vi "Stop.vi"(8 "error in (no error)":errorcluster, 11 "Monitor in":refnum<class "Monitor.lvclass">) -> (0 "error out":errorcluster, 3 "Monitor out":refnum<class "Monitor.lvclass">)   [LabVIEW 2016, in "Monitor.lvclass"]
uses:
  Monitor.lvclass
  Command/Command.lvclass
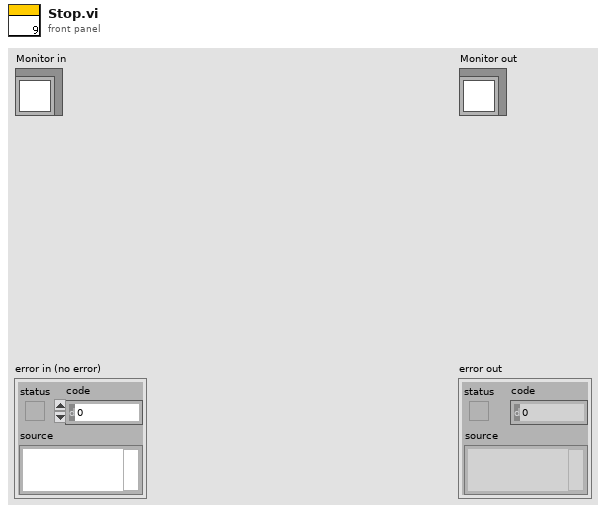
[diagram p1: front panel]
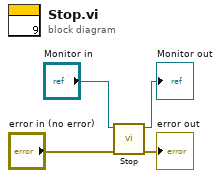
[diagram p0: block diagram]
diagram:
  n1 = call-parent "Stop.vi"("error in (no error)"="error in (no error)", "Command in"="Monitor in") -> ("error out"=→"error out":errorcluster, "Command out"=→"Monitor out":refnum<class "Monitor.lvclass">)  [unwired: 8 in]
